vi "4.6.2.vi"() -> ()   [LabVIEW 2018]
uses:
  <vilib>/Analysis/baseanly.llb/Mean (DBL).vi
  <vilib>/Analysis/NI_AALBase.lvlib
panel:
  out "병아리반 토익 평균 2":dbl
  out "병아리반 토익 평균":dbl
  in  "병아리반":cluster{"문자열":string, "숫자형":dbl, "불리언":bool}[](array[cluster])
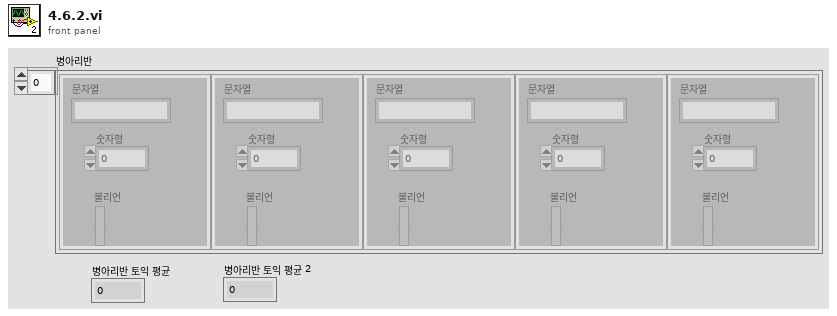
[diagram p1: front panel]
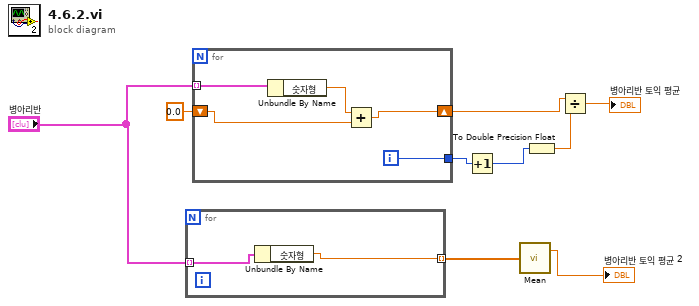
[diagram p0: block diagram]
diagram:
  n1 = for {
    tunnel: "병아리반" -> [w11] mode=indexing
    tunnel: [w10] -> w7 mode=indexing
    n2 = Unbundle By Name(w11) -> ("숫자형"=w10:dbl)
  }
  n3 = for {
    shift-right: [w13] -> w5
    shift-left: 0.0 -> [w14]
    tunnel: "병아리반" -> [w16] mode=indexing
    tunnel: [w12] -> w4
    i -> [w12]
    n4 = Unbundle By Name(w16) -> ("숫자형"=w15:dbl)
    n5 = Add(x=w15, y=w14) -> (x+y=w13:dbl)
  }
  n6 = Increment(x=w4) -> (x+1=w3:i32)
  n7 = call-poly <vilib>:"Mean.vi"("X"=w7) -> ("mean"=→"병아리반 토익 평균 2":dbl)  [unwired: 1 out]
  n8 = To Double Precision Float(number=w3) -> (double precision float=w2:dbl)
  n9 = Divide(x=w5, y=w2) -> (x/y=→"병아리반 토익 평균":dbl)
